vi "Save Test Information.vi"(8 "error in (no error)":errorcluster, 10 "Test Information":T1, 11 "csv-formatter in":refnum<class "csv-formatter.lvclass">) -> (0 "error out":errorcluster, 3 "csv-formatter out":refnum<class "csv-formatter.lvclass">)   [LabVIEW 2015, in "csv-formatter.lvclass"]
doc: "This VI will save the DUT Information to the permanent report"
uses:
  csv-formatter.lvclass
  Report Information/Test Information.ctl
  csv-formatter.lvclass/csv-formatter.ctl
  Report Information/Report Information.lvclass
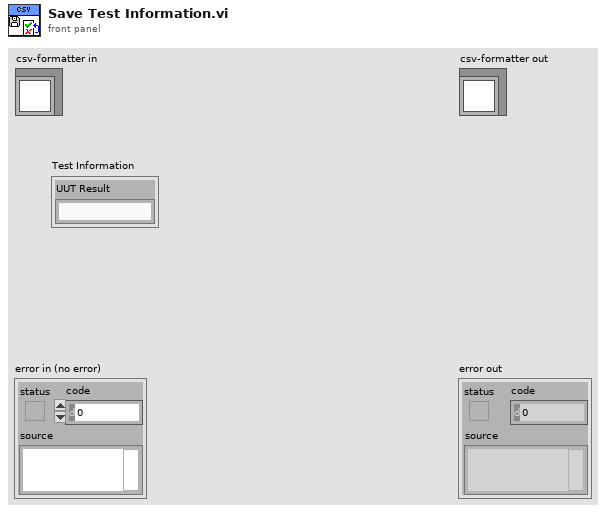
[diagram p1: front panel]
types:
  T1 = typedef "Report Information.lvclass/Test Information.ctl" = cluster{"UUT Result":string}
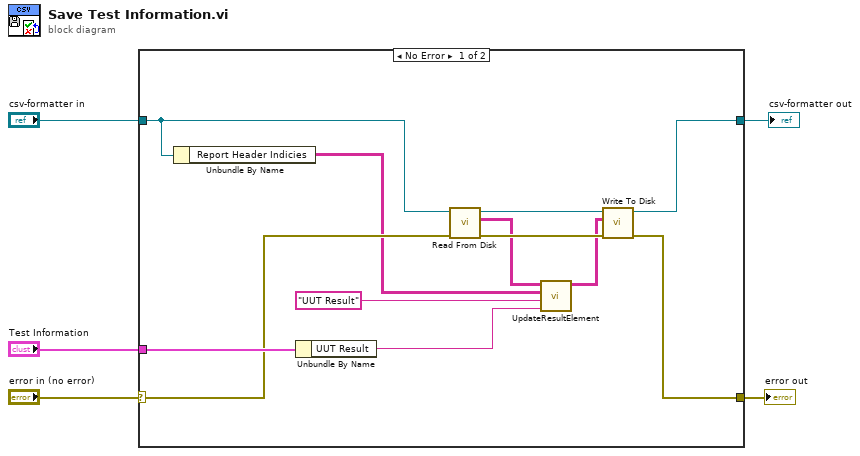
[diagram p0: block diagram]
diagram:
  n1 = case shown="No Error" "error in (no error)" {
    selector: "error in (no error)" -> [w16 w19]
    tunnel: "Test Information" -> [w17 _]
    tunnel: "csv-formatter in" -> [w10 w18]
    tunnel: [w14 w19] -> w2
    tunnel: [w8 w18] -> w1
    frame No Error {
      n2 = Unbundle By Name(w10) -> ("Report Header Indicies"=w12:string[][])
      n3 = Unbundle By Name(w17) -> ("UUT Result"=w6:string)
      n4 = call "Read From Disk.vi"("error in (no error)"=w16, "csv-formatter in"=w10) -> ("error out"=w15:errorcluster, "Result Out"=w11:string[][], "csv-formatter out"=w9:refnum<class "csv-formatter.lvclass">)  [unwired: 7 in]
      n5 = call "UpdateResultElement.vi"("Data"=w6, "Lookup String"="UUT Result", "Report Header Indicies in"=w12, "Result in"=w11) -> ("Result Out"=w13:string[][])  [unwired: 6 in, 1 out]
      n6 = call "Write To Disk.vi"("error in (no error)"=w15, "Result In"=w13, "csv-formatter in"=w9) -> ("error out"=w14:errorcluster, "csv-formatter out"=w8:refnum<class "csv-formatter.lvclass">)  [unwired: 7 in]
    }
    frame Error {
    }
  }
  "error out" <- w2
  "csv-formatter out" <- w1
